vi "comm break.vi"(8 "error in (no error)":errorcluster, 10 "Milliseconds":u32, 11 "Comm Handle":u32) -> (0 "error out":errorcluster, 3 "dup Comm Handle":u32)   [LabVIEW 2017, in "lvserial.lvlib"]
doc: "This function suspends character transmission for a specified communications device and places the transmission line in a break state for x milliseconds. Afterwards this VI restores character transmission for a specified communications device and places the transmission line in a nonbreak state."
uses:
  lvserial.lvlib
  lvserial.dll
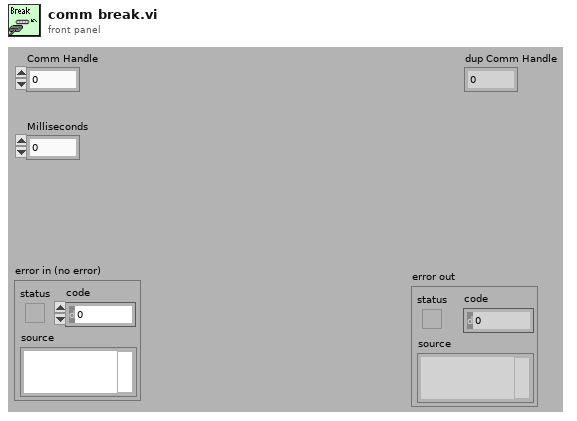
[diagram p1: front panel]
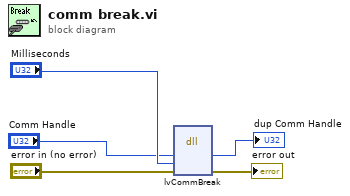
[diagram p0: block diagram]
diagram:
  n1 = dll-call lib="lvserial.dll" fn="lvCommBreak"("hComm"="Comm Handle", "ulMilliseconds"="Milliseconds", "error in (no error)"="error in (no error)") -> ("hComm"=→"dup Comm Handle":u32, "error in (no error)"=→"error out":errorcluster)  [unwired: 4 in, 3 out]
